vi "SIM_CurrentOutput.vi"(9 "array":dbl[][](array[numeric]), 10 "?":cluster{"x (m)":dbl, "y (m)":dbl, "z (mm)":dbl} {"z (mm)" format="%.1f"; "y (m)" format="%.1p"; "x (m)" format="%.1p"}) -> (3 "Current Out (A)":dbl, 4 "Zread":dbl)   [LabVIEW 2017]
uses:
  <vilib>/ptbypt/NI_PtbyPt.lvlib
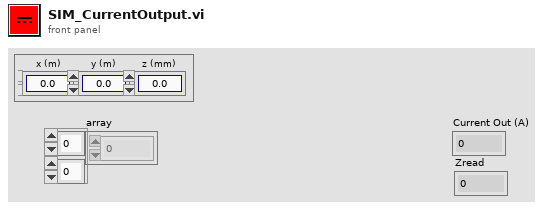
[diagram p1: front panel]
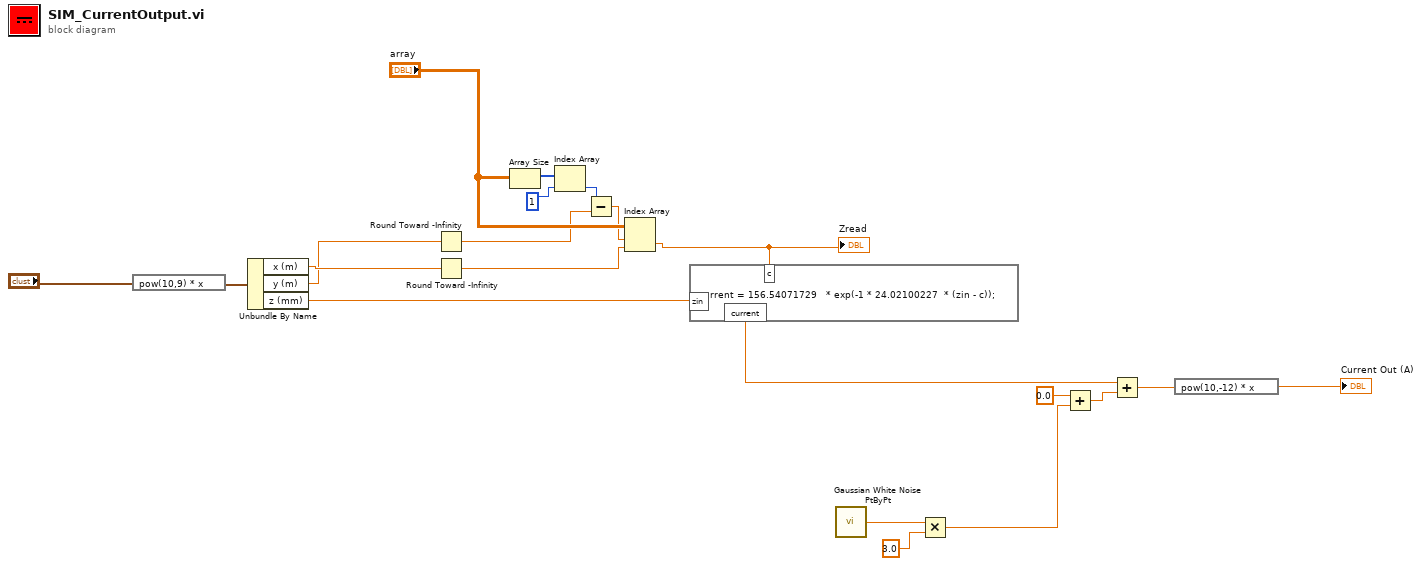
[diagram p0: block diagram]
diagram:
  n1 = expression code="pow(10,9) * x"("?") -> (w12:cluster{"x (m)":dbl, "y (m)":dbl, "z (mm)":dbl})
  n2 = Unbundle By Name(w12) -> ("x (m)"=w11:dbl, "y (m)"=w10:dbl, "z (mm)"=w9:dbl)
  n3 = Round Toward -Infinity(1:w10) -> (0:w1:dbl)
  n4 = Round Toward -Infinity(1:w11) -> (0:w21:dbl)
  n5 = Array Size(array="array") -> (size(s)=w5:i32[])
  n6 = Index Array(array=w5, index=1) -> (element=w2:i32)
  n7 = Subtract(x=w2, y=w1) -> (x-y=w3:dbl)
  n8 = Index Array(array="array", index (row)=w3, index (col)=w21) -> (element=w14:dbl)
  "Zread" <- w14
  n9 = formula code="current = 156.54071729   * exp(-1 * 24.02100227  * (zin - c));"("zin"=w9, "c"=w14) -> ("current"=w15:dbl)
  n10 = call <vilib>:"Gaussian White Noise PtByPt.vi"() -> ("Gaussian white noise"=w20:dbl)  [unwired: 3 in]
  n11 = Multiply(x=w20, y=3.0) -> (x*y=w17:dbl)
  n12 = Add(x=0.0, y=w17) -> (x+y=w18:dbl)
  n13 = Add(x=w15, y=w18) -> (x+y=w8:dbl)
  n14 = expression code="pow(10,-12) * x"(w8) -> (→"Current Out (A)":dbl)
